vi "String_Facade.vi"(0 "Data In":T5, 2 "Display State In":T2, 3 "Container State":T4) -> (6 "Data Out":T5, 7 "Display State Out":T2, 8 "Action":T1)   [LabVIEW 2012, in "String_XControl.xctl"]
uses:
  String_XControl.xctl
  String_Data.ctl
  <vilib>/_xctls/Container State.ctl
  String_State.ctl
  <vilib>/Utility/miscctls.llb/LVFontTypeDef.ctl
  <vilib>/_xctls/Action.ctl
  <vilib>/_xctls/XControlSupport.lvlib
panel:
  in  "Length":i32=10
  in  "String":string
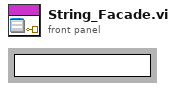
[diagram p1: front panel]
types:
  T1 = typedef "XControlSupport.lvlib/Action.ctl" = cluster{"Data Changed?":bool, "State Changed?":bool, "Action Name":string}
  T2 = typedef "String_XControl.xctl/String_State.ctl" = cluster{"String Length":i32, "Font":T3}
  T3 = typedef "LVFontTypeDef.ctl" = cluster{"Font Name":string, "Size":u16, "Bold":bool, "Italic":bool, "Underline":bool, "Strikeout":bool, "Color":u32}
  T4 = typedef "XControlSupport.lvlib/Container State.ctl" = cluster{"Indicator?":bool, "Run Mode?":bool, " Refnum":refnum<vi>}
  T5 = typedef "String_XControl.xctl/String_Data.ctl" = string
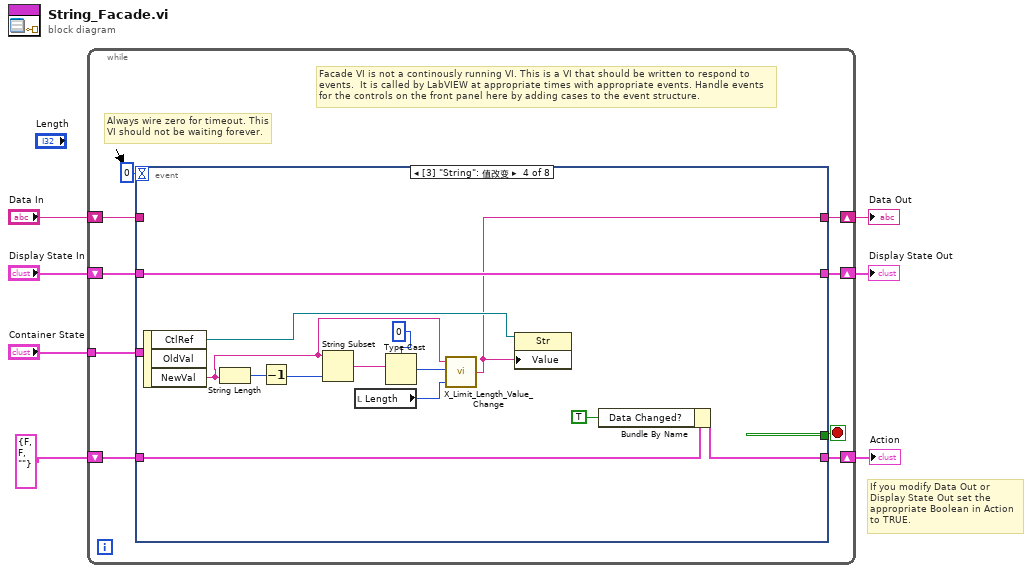
[diagram p0: block diagram]
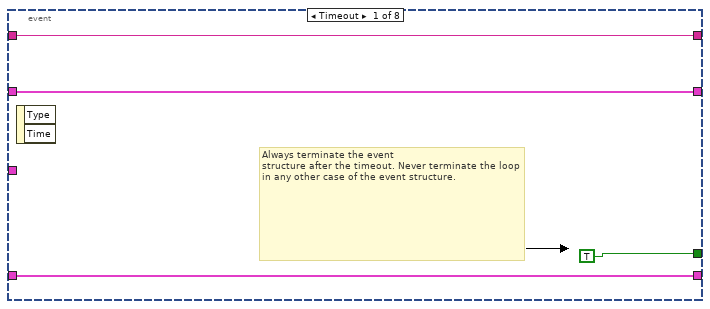
[diagram p2: hidden frame]
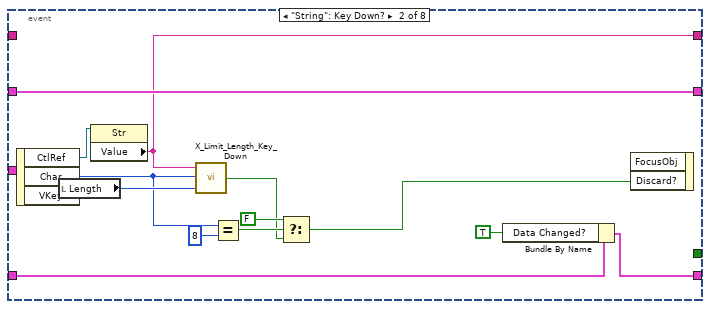
[diagram p3: hidden frame]
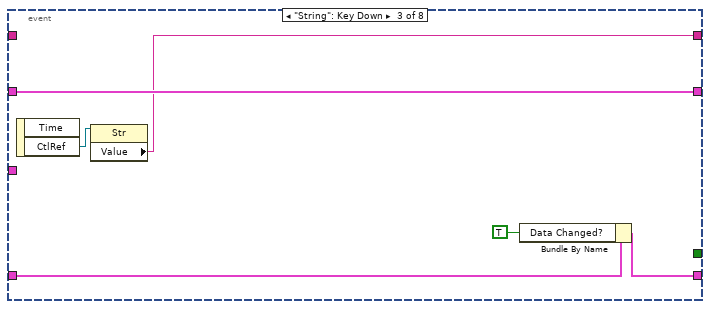
[diagram p4: hidden frame]
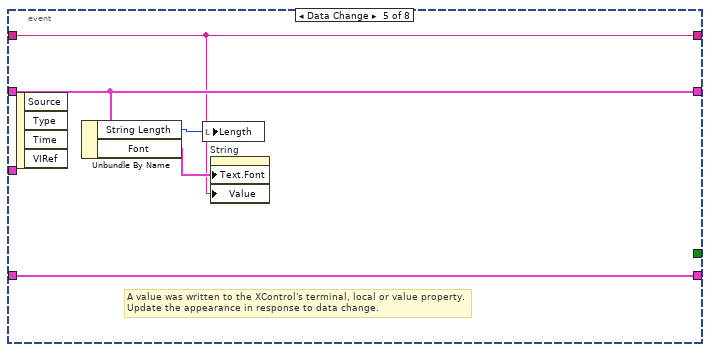
[diagram p5: hidden frame]
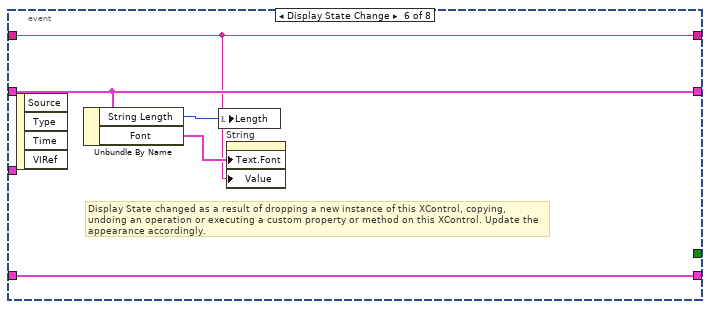
[diagram p6: hidden frame]
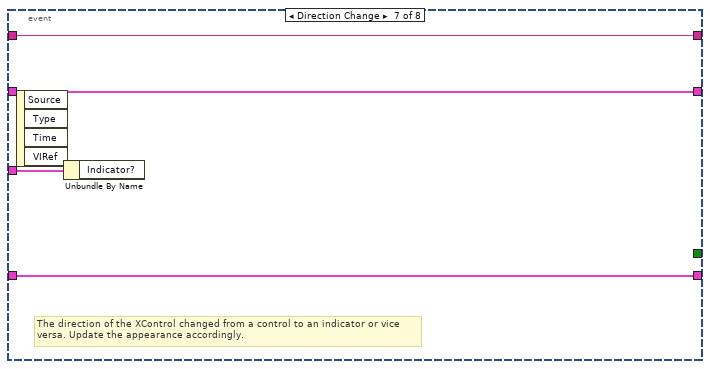
[diagram p7: hidden frame]
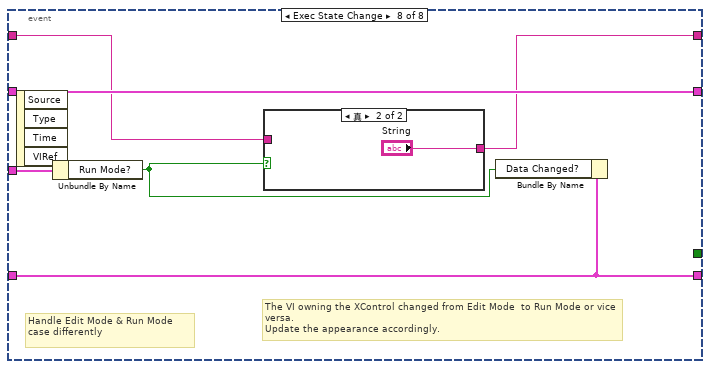
[diagram p8: hidden frame]
diagram:
  # "If you modify Data Out or\nDisplay State Out set the\nappropriate Boolean in Action\nto TRUE."
  n1 = while {
    shift-right: [w15] -> w4
    shift-left: "Display State In" -> [w16]
    tunnel: "Container State" -> [w12]
    shift-right: [w10] -> w7
    shift-left: "Data In" -> [w11]
    shift-right: [w8] -> w2
    shift-left: T1 {"Data Changed?"=FALSE, "State Changed?"=FALSE, "Action Name"=""} ("Action") -> [w9]
    stop <- w14 stop-if-true
    # "Facade VI is not a continously running VI. This is a VI that should be written to respond to events.  It is called by LabVIEW at appropriate times with appropriate events. Handle events for the controls on the front panel here by adding cases to the event structure."
    # "Always wire zero for timeout. This\nVI should not be waiting forever."
    n2 = event shown="[3] \"String\": 值改变" {
      selector: _ -> [_ _ _ _ _ _ _ _]
      dyn-events: _ -> [_ _ _ _ _ _ _ _]
      timeout: 0 -> [_ _ _ _ _ _ _ _]
      tunnel: w16 -> [w18 w33 w39 w52 w56 w61 w65 w71]
      tunnel: [w18 w33 w39 w52 w56 w61 w65 w71] -> w15
      tunnel: [TRUE _ _ _ _ _ _ _] -> w14
      tunnel: w12 -> [_ _ _ _ _ _ w66 w72]
      tunnel: w11 -> [w17 _ _ _ w53 w58 w64 w68]
      tunnel: [w17 w30 w37 w43 w53 w58 w64 w67] -> w10
      tunnel: [w19 w27 w34 w41 w57 w62 w63 w70] -> w8
      tunnel: w9 -> [w19 w28 w35 w42 w57 w62 w63 w70]
      event Timeout {
        # "Always terminate the event\nstructure after the timeout. Never terminate the loop in any other case of the event structure."
        n3 = event-data() -> ()  [unwired: 3 out]
      }
      event "String": Key Down? {
        n4 = event-data() -> ("CtlRef"=w32:refnum<vi>, "Char"=w26:i16)  [unwired: 2 out]
        n5 = local read "Length"() -> (w31:i32)
        n6 = property class="Str"(reference=w32) -> ("Value"=w30:string)  [unwired: 1 in, 2 out]
        n7 = call "X_Limit_Length_Key_Down.vi"("Max String Length"=w31, "Char"=w26, "Input String"=w30) -> ("Discard?"=w22:bool)
        n8 = Equal?(x=w26, y=i16 8) -> (x = y?=w24:bool)
        n9 = Select(t=FALSE, s=w24, f=w22) -> (s? t:f=w21:bool)
        n10 = Bundle By Name(cluster=w28, "Data Changed?"=TRUE) -> (w27:T1)
        n11 = event-data("Discard?"=w21) -> ()  [unwired: 1 in, 2 out]
      }
      event "String": Key Down {
        n12 = event-data() -> ("CtlRef"=w38:refnum<vi>)  [unwired: 2 out]
        n13 = property class="Str"(reference=w38) -> ("Value"=w37:string)  [unwired: 1 in, 2 out]
        n14 = Bundle By Name(cluster=w35, "Data Changed?"=TRUE) -> (w34:T1)
      }
      event "String": Value Change {
        n15 = event-data() -> ("CtlRef"=w44:refnum<vi>, "NewVal"=w45:string)  [unwired: 2 out]
        n16 = String Length(string=w45) -> (length=w51:i32)
        n17 = Decrement(x=w51) -> (x-1=w50:i32)
        n18 = String Subset(string=w45, length (rest)=w50) -> (substring=w49:string)  [unwired: 1 out]
        n19 = local read "Length"() -> (w46:i32)
        n20 = Type Cast(type=i16 0, x=w49) -> (*(type *) &x=w47:i16)
        n21 = call "X_Limit_Length_Value_Change.vi"("Max String Length"=w46, "Char"=w47, "Input String"=w45) -> ("Result String"=w43:string)
        n22 = property class="Str"(reference=w44, "Value"=w43) -> ()  [unwired: 1 in, 2 out]
        n23 = Bundle By Name(cluster=w42, "Data Changed?"=TRUE) -> (w41:T1)
      }
      event Data Change {
        # "A value was written to the XControl's terminal, local or value property.\nUpdate the appearance in response to data change."
        n24 = event-data() -> ()  [unwired: 5 out]
        n25 = Unbundle By Name(w56) -> ("String Length"=w55:i32, "Font"=w54:T3)
        n26 = local write "Length"(w55) -> ()
        n27 = property on="String" class="Str"("Text.Font"=w54, "Value"=w53) -> ()  [unwired: 2 in, 2 out]
      }
      event Display State Change {
        # "Display State changed as a result of dropping a new instance of this XControl, copying, undoing an operation or executing a custom property or method on this XControl. Update the appearance accordingly."
        n28 = event-data() -> ()  [unwired: 5 out]
        n29 = Unbundle By Name(w61) -> ("String Length"=w60:i32, "Font"=w59:T3)
        n30 = local write "Length"(w60) -> ()
        n31 = property on="String" class="Str"("Text.Font"=w59, "Value"=w58) -> ()  [unwired: 2 in, 2 out]
      }
      event Direction Change {
        # "The direction of the XControl changed from a control to an indicator or vice versa. Update the appearance accordingly."
        n32 = event-data() -> ()  [unwired: 5 out]
        n33 = Unbundle By Name(w66) -> ()  [unwired: 1 out]
      }
      event Exec State Change {
        # "The VI owning the XControl changed from Edit Mode  to Run Mode or vice versa.\nUpdate the appearance accordingly."
        # "Handle Edit Mode & Run Mode\ncase differently"
        n34 = event-data() -> ()  [unwired: 5 out]
        n35 = Unbundle By Name(w72) -> ("Run Mode?"=w69:bool)
        n36 = case shown="真" w69 {
          tunnel: w68 -> [w73 _]
          tunnel: [w73 "String"] -> w67
          frame False {
          }
          frame True {
          }
        }
        n37 = Bundle By Name(cluster=w70, "Data Changed?"=w69) -> ()  [unwired: 1 out]
      }
    }
  }
  "Display State Out" <- w4
  "Data Out" <- w7
  "Action" <- w2
